vi "PH_Beckhoff_10BB_Plus.declare Tags.vi"(2 "error in (no error)":errorcluster, 3 "Instance Name":string) -> (0 "error out":errorcluster, 1 "Data in cluster":T1={"Default Values"={"Sonderklemmen Inputs"=[], "Analog Inputs"=[], "Analog Outputs"=[], "Digital Inputs"=[], "Digital Outputs"=[]}, "Description"="", "Hardware configured?"=TRUE, "Activate Change Manager?"=FALSE, "Difference to handle an analog input as change"=1})   [LabVIEW 2014, in "PH_Beckhoff_10BB_Plus.lvlib"]
doc: "This VI declares the tagnames and sets the scaling of the tags of this class."
uses:
  PH_Beckhoff_10BB_Plus.lvlib
  PH_Beckhoff/PH_Beckhoff.constructor Data in.ctl
  PH_Beckhoff/PH_Beckhoff.Values.ctl
  PH_Beckhoff/PH_Beckhoff.Sonderklemmen Inputs.ctl
  PH_Beckhoff/PH_Beckhoff.Analog Inputs.ctl
  PH_Beckhoff/PH_Beckhoff.Scaling Type.ctl
  PH_Beckhoff/PH_Beckhoff.Analog Outputs.ctl
  PH_Beckhoff/PH_Beckhoff.Digital Inputs.ctl
  PH_Beckhoff/PH_Beckhoff.Digital Outputs.ctl
  PH_Beckhoff/PH_Beckhoff.lvlib
  PH_Basics/PH_Common/PH_Common.lvlib
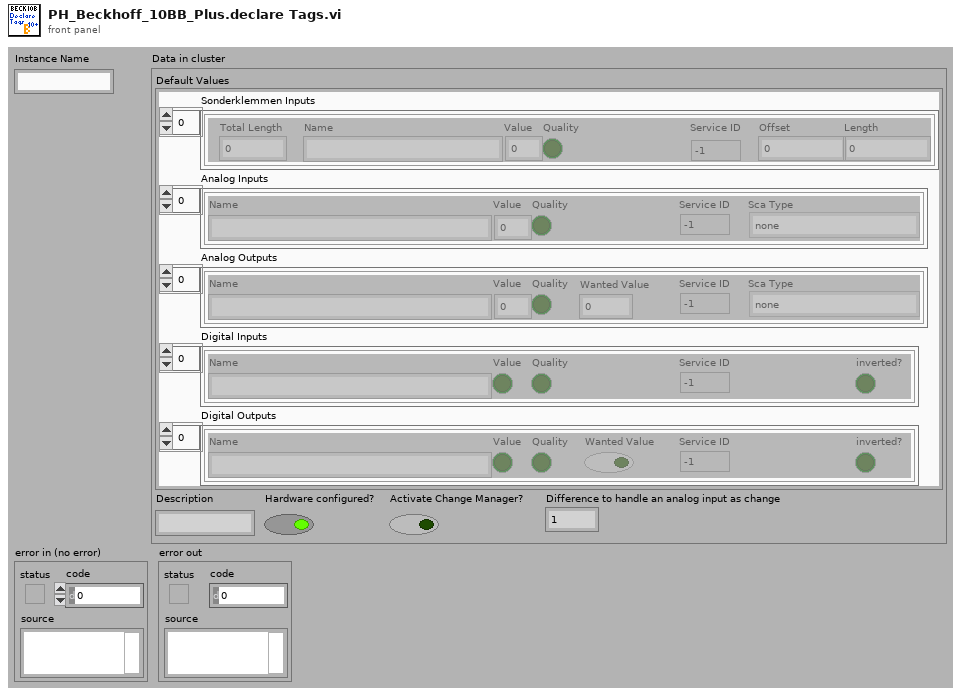
[diagram p1: front panel]
types:
  T1 = typedef "PH_Beckhoff.lvlib/PH_Beckhoff.constructor Data in.ctl" = cluster{"Default Values":T2, "Description":string, "Hardware configured?":bool, "Activate Change Manager?":bool, "Difference to handle an analog input as change":u32}
  T2 = typedef "PH_Beckhoff.lvlib/PH_Beckhoff.Values.ctl" = cluster{"Sonderklemmen Inputs":T3, "Analog Inputs":T4, "Analog Outputs":T6, "Digital Inputs":T7, "Digital Outputs":T8}
  T3 = typedef "PH_Beckhoff.lvlib/PH_Beckhoff.Sonderklemmen Inputs.ctl" = cluster{"Total Length":u32, "Name":string, "Value":u64, "Quality":bool, "Service ID":i32, "Offset":u32, "Length":u32}[]
  T4 = typedef "PH_Beckhoff.lvlib/PH_Beckhoff.Analog Inputs.ctl" = cluster{"Name":string, "Value":u32, "Quality":bool, "Service ID":i32, "Sca Type":T5}[]
  T5 = typedef "PH_Beckhoff.lvlib/PH_Beckhoff.Scaling Type.ctl" = enum16{"none", "0 ... 15 Bit -> 0 ... 5", "0 ... 15 Bit -> 0 ... 10", "0 ... 15 Bit -> 0 ... 25", "0 ... 15 Bit -> 4 ... 20", "0 ... 15 Bit -> 0 ... 1", "0 ... 15 Bit -> 0 ... 20000", "0 ... 15 Bit -> 0 ... 24000"}
  T6 = typedef "PH_Beckhoff.lvlib/PH_Beckhoff.Analog Outputs.ctl" = cluster{"Name":string, "Value":u32, "Quality":bool, "Wanted Value":u32, "Service ID":i32, "Sca Type":T5}[]
  T7 = typedef "PH_Beckhoff.lvlib/PH_Beckhoff.Digital Inputs.ctl" = cluster{"Name":string, "Value":bool, "Quality":bool, "Service ID":i32, "inverted?":bool}[]
  T8 = typedef "PH_Beckhoff.lvlib/PH_Beckhoff.Digital Outputs.ctl" = cluster{"Name":string, "Value":bool, "Quality":bool, "Wanted Value":bool, "Service ID":i32, "inverted?":bool}[]
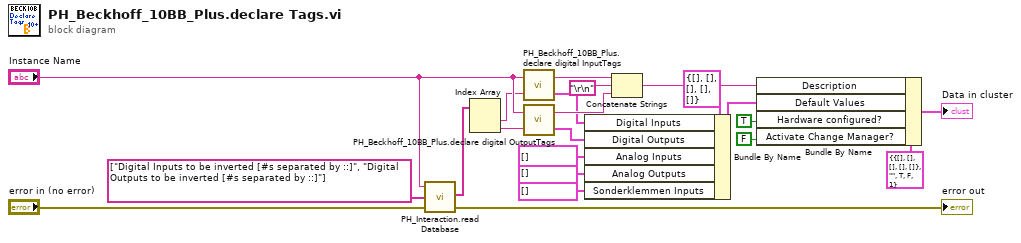
[diagram p0: block diagram]
diagram:
  n1 = call "PH_Interaction.read Database.vi"("error in (no error)"="error in (no error)", "Strings to search for"=string[] ["Digital Inputs to be inverted [#s separated by ::]", "Digital Outputs to be inverted [#s separated by ::]"] ("Strings to search for in"), "DB Entry to read"="Instance Name") -> ("error out"=→"error out":errorcluster, "Values"=w4:string[])  [unwired: 1 in]
  n2 = Index Array(array=w4) -> (element #1=w3:string, element #2=w2:string)  [unwired: 2 in]
  n3 = call "PH_Beckhoff_10BB_Plus.declare digital InputTags.vi"("Digital Inputs to be inverted [#s separated by ::]"=w3, "Instance Name"="Instance Name") -> ("Digital Inputs"=w10:T7, "Description"=w16:string)
  n4 = call "PH_Beckhoff_10BB_Plus.declare digital OutputTags.vi"("Outputs to be inverted [#s separated by ::]"=w2, "Instance Name"="Instance Name") -> ("Digital Outputs"=w11:T8, "Description"=w15:string)
  n5 = Bundle By Name(cluster=T2 {"Sonderklemmen Inputs"=[], "Analog Inputs"=[], "Analog Outputs"=[], "Digital Inputs"=[], "Digital Outputs"=[]} ("Dummy Default Values"), "Digital Inputs"=w10, "Digital Outputs"=w11, "Analog Inputs"=T4 [], "Analog Outputs"=T6 [], "Sonderklemmen Inputs"=T3 []) -> (w18:T2)
  n6 = Concatenate Strings(w16, "\r\n", w15) -> (w14:string)
  n7 = Bundle By Name(cluster=T1 {"Default Values"={"Sonderklemmen Inputs"=[], "Analog Inputs"=[], "Analog Outputs"=[], "Digital Inputs"=[], "Digital Outputs"=[]}, "Description"="", "Hardware configured?"=TRUE, "Activate Change Manager?"=FALSE, "Difference to handle an analog input as change"=1} ("Dummy data in cluster"), "Description"=w14, "Default Values"=w18, "Hardware configured?"=TRUE, "Activate Change Manager?"=FALSE) -> (→"Data in cluster":T1)
